vi "PH_USB600x_AnalogReader.ProcCases.vi"(0 "i ref in":refnum<vi>, 1 "selector":string, 2 "Data":T1, 3 "call cluster":T2={"Object"="", "Selector"="", "CallType"=enum."synchronous", "Async Object"="", "Async Selector"="", "Data Descriptor"="", "Data"=[], "Error #"=0, "Expire"=0}, 5 "error in (no error)":errorcluster) -> (14 "i ref out":refnum<vi>, 17 "answer cluster":T2={"Object"="", "Selector"="", "CallType"=enum."synchronous", "Async Object"="", "Async Selector"="", "Data Descriptor"="", "Data"=[], "Error #"=0, "Expire"=0}, 19 "error out":errorcluster)   [LabVIEW 2014, in "PH_USB600x_AnalogReader.lvlib"]
doc: "This method is called by a process from within the default case in the event loop. The methods of a class that are linked to events will be called from THIS method. Add your code here."
uses:
  PH_USB600x_AnalogReader.lvlib
  CS_Core/CSSystem/CoreDefs/CoreDefs.call_type.ctl
  CS_Core/BaseProcess/BaseProcess.descriptor string definition.ctl
  CS_Core/CSSystem/CoreDefs/CoreDefs.rawDataType.ctl
  CS_Core/CSSystem/CoreLib/CoreLib.byte array 2 int.vi
  CS_Core/CSSystem/CoreLib/CoreLib.byte array 2 double.vi
  CS_Core/CSSystem/CoreLib/CoreLib.string 2 byte array.vi
  CS_Core/CSSystem/CoreLib/CoreLib.byte array 2 string.vi
  CS_Core/CSSystem/CoreLib/CoreLib.byte array 2 short.vi
  CS_Core/CSSystem/CoreLib/CoreLib.lvlib
  CS_Core/BaseProcess/BaseProcess.lvlib
  CS_Core/CSApplicationBaseClasses/DeviceBase/DeviceBase.lvlib
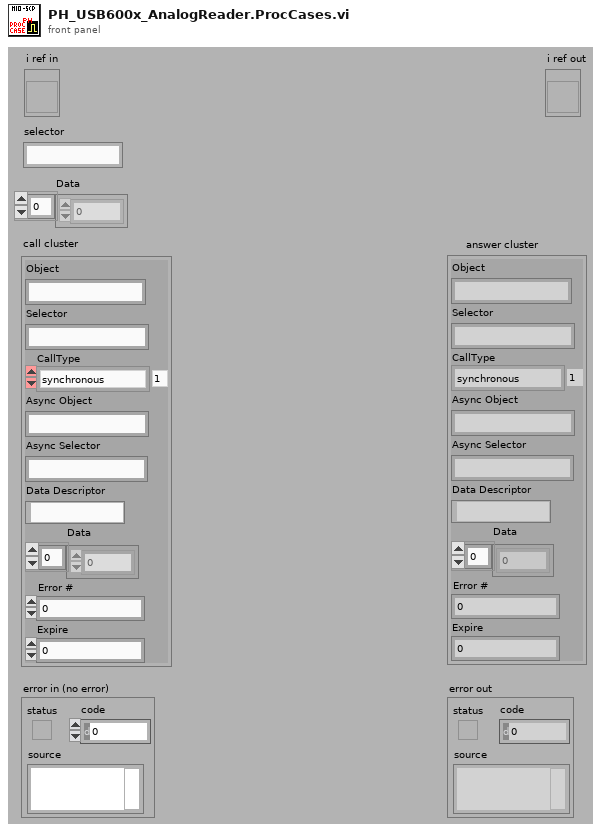
[diagram p1: front panel]
types:
  T1 = typedef "CoreDefs.rawDataType.ctl" = i8[]
  T2 = typedef "CoreDefs.call_type.ctl" = cluster{"Object":string, "Selector":string, "CallType":enum16{"simple", "synchronous", "asynchronous"}, "Async Object":string, "Async Selector":string, "Data Descriptor":T3, "Data":T1, "Error #":i32, "Expire":u32}
  T3 = typedef "BaseProcess.lvlib/BaseProcess.descriptor string definition.ctl" = string
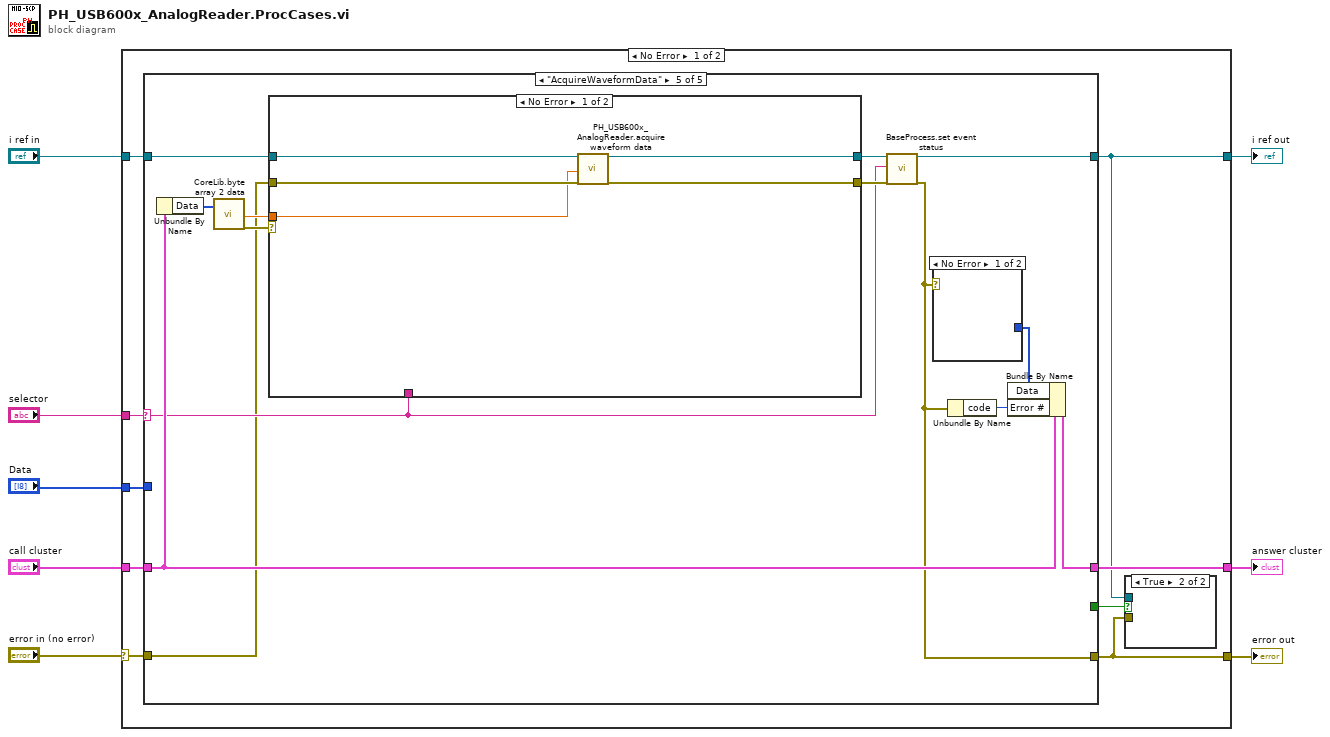
[diagram p0: block diagram]
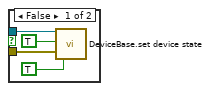
[diagram p2: hidden frame]
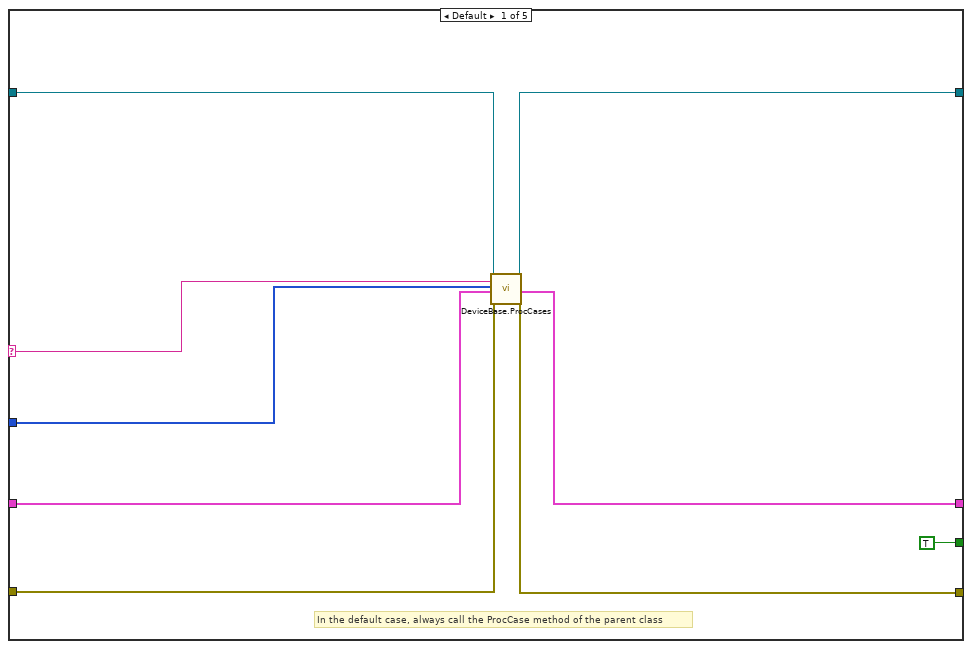
[diagram p3: hidden frame]
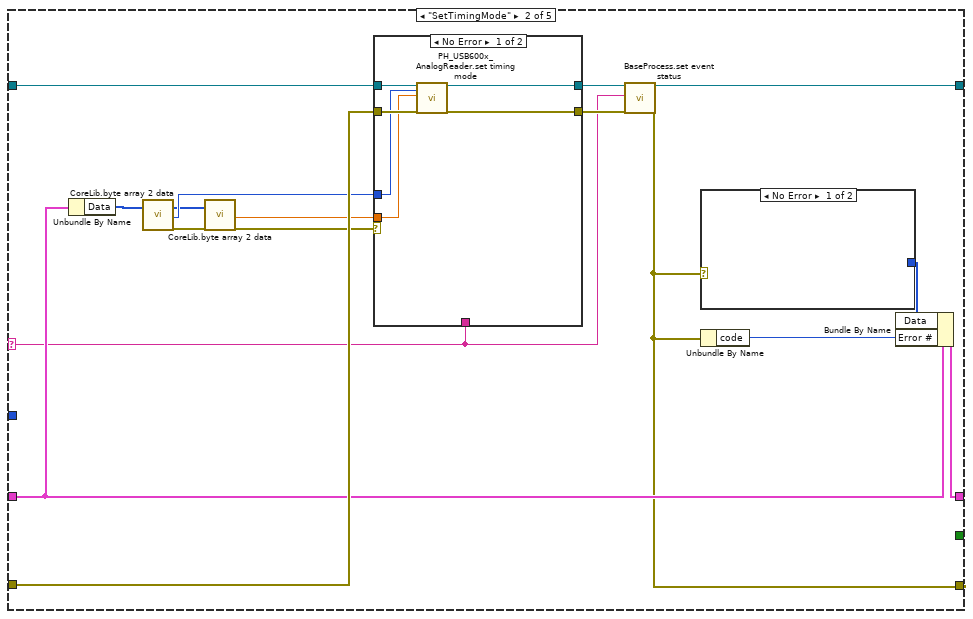
[diagram p4: hidden frame]
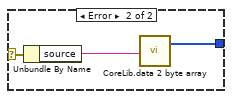
[diagram p5: hidden frame]
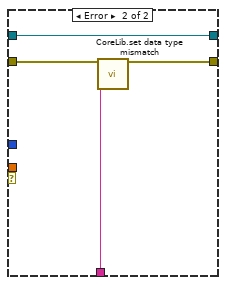
[diagram p6: hidden frame]
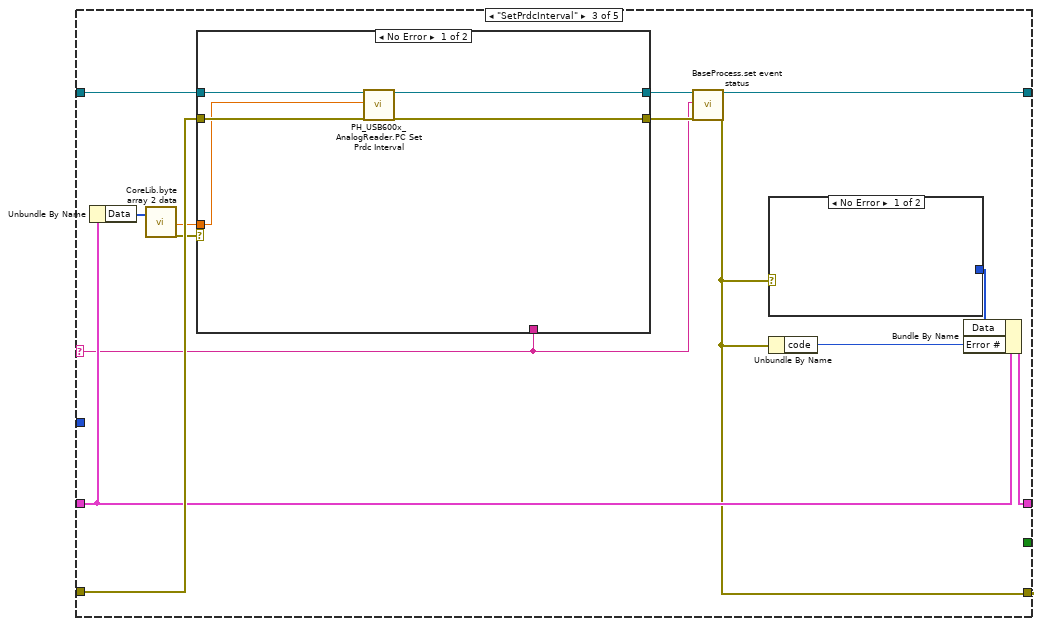
[diagram p7: hidden frame]
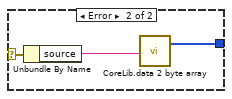
[diagram p8: hidden frame]
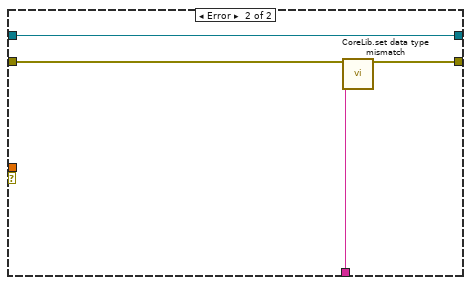
[diagram p9: hidden frame]
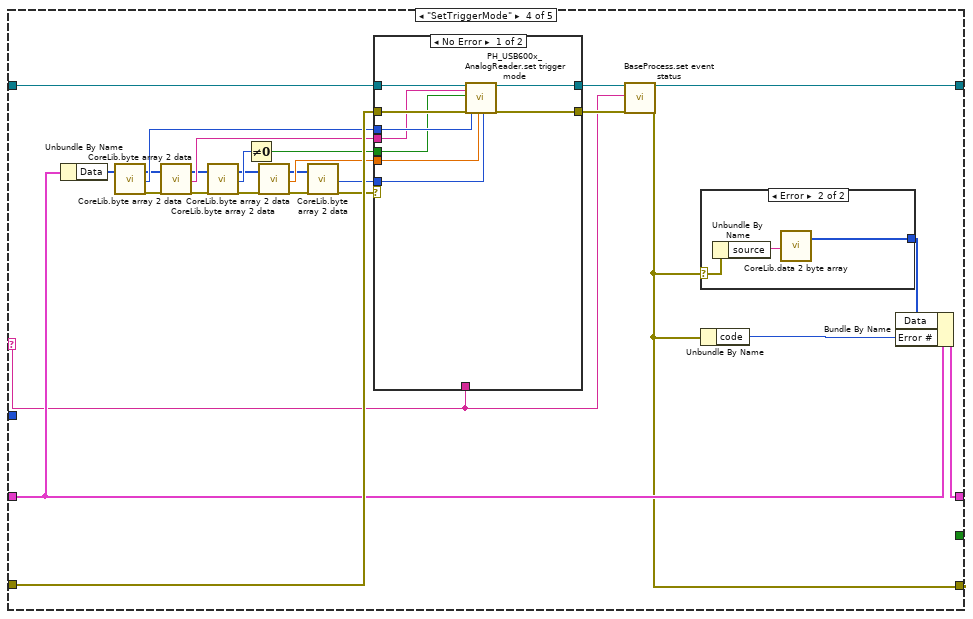
[diagram p10: hidden frame]
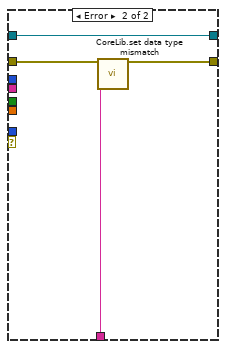
[diagram p12: hidden frame]
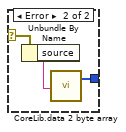
[diagram p13: hidden frame]
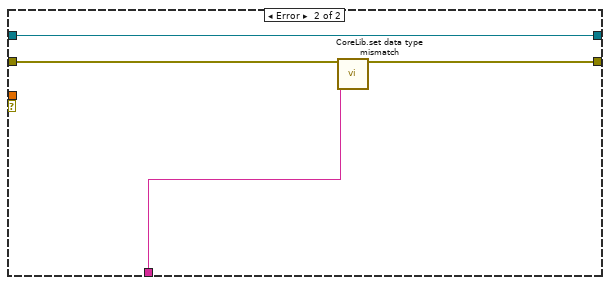
[diagram p14: hidden frame]
diagram:
  n1 = case shown="No Error" "error in (no error)" {
    selector: "error in (no error)" -> [w12 w156]
    tunnel: "selector" -> [w17 _]
    tunnel: [w16 w157] -> w7
    tunnel: "Data" -> [w15 _]
    tunnel: "call cluster" -> [w14 w157]
    tunnel: "i ref in" -> [w13 w158]
    tunnel: [w10 w158] -> w3
    tunnel: [w9 w156] -> w2
    frame No Error {
      n2 = case shown="\"AcquireWaveformData\"" w17 {
        selector: w17 -> [w24 w38 w65 w104 w135]
        tunnel: w15 -> [w25 _ _ _ _]
        tunnel: w13 -> [w23 w47 w74 w113 w143]
        tunnel: [w30 w37 w64 w103 w134] -> w10
        tunnel: w14 -> [w26 w44 w71 w110 w141]
        tunnel: [w27 w43 w70 w109 w140] -> w16
        tunnel: w12 -> [w29 w46 w73 w112 w130]
        tunnel: [w28 w39 w66 w105 w136] -> w9
        tunnel: [TRUE _ _ _ _] -> w11
        frame Default {
          # "In the default case, always call the ProcCase method of the parent class"
          n3 = call "DeviceBase.ProcCases.vi"("i ref in"=w23, "selector"=w24, "Data"=w25, "call cluster"=w26, "error in (no error)"=w29) -> ("i ref out"=w30:refnum<vi>, "answer cluster"=w27:T2, "error out"=w28:errorcluster)  [unwired: 12 in]
        }
        frame "SetTimingMode" {
          n4 = Unbundle By Name(w44) -> ("Data"=w36:T1)
          n5 = call-poly "CoreLib.byte array 2 data.vi"("byteArray"=w36) -> ("byteArray out"=w34:T1, "i32"=w35:i32, "error out"=w32:errorcluster)  [unwired: 16 in]
          n6 = call-poly "CoreLib.byte array 2 data.vi"("byteArray"=w34, "error in (no error)"=w32) -> ("d64"=w33:dbl, "error out"=w31:errorcluster)  [unwired: 15 in, 1 out]
          n7 = case shown="No Error" w31 {
            tunnel: [w51 w60] -> w41
            tunnel: w47 -> [w56 w60]
            tunnel: w46 -> [w55 w59]
            tunnel: [w52 w58] -> w40
            tunnel: w33 -> [w53 _]
            tunnel: w38 -> [_ w57]
            tunnel: w35 -> [w54 _]
            frame No Error {
              n8 = call "PH_USB600x_AnalogReader.set timing mode.vi"("i ref in"=w56, "Samples per Channel"=w54, "Rate"=w53, "error in (no error)"=w55) -> ("i ref out"=w51:refnum<vi>, "error out"=w52:errorcluster)  [unwired: 14 in]
            }
            frame Error {
              n9 = call "CoreLib.set data type mismatch.vi"("error in (no error)"=w59, "error source"=w57) -> ("error out"=w58:errorcluster)  [unwired: 17 in]
            }
          }
          n10 = call "BaseProcess.set event status.vi"("i ref in"=w41, "EventStatus"=w38, "error in (no error)"=w40) -> ("i ref out"=w37:refnum<vi>, "error out"=w39:errorcluster)  [unwired: 14 in, 1 out]
          n11 = case shown="No Error" w39 {
            selector: w39 -> [_ w50]
            tunnel: [_ w48] -> w42
            frame No Error {
            }
            frame Error {
              n12 = Unbundle By Name(w50) -> ("source"=w49:string)
              n13 = call-poly "CoreLib.data 2 byte array.vi"("string"=w49) -> ("byteArray out"=w48:T1)  [unwired: 18 in]
            }
          }
          n14 = Unbundle By Name(w39) -> ("code"=w45:i32)
          n15 = Bundle By Name(cluster=w44, "Data"=w42, "Error #"=w45) -> (w43:T2)
        }
        frame "SetPrdcInterval" {
          n16 = Unbundle By Name(w71) -> ("Data"=w61:T1)
          n17 = call-poly "CoreLib.byte array 2 data.vi"("byteArray"=w61) -> ("d64"=w63:dbl, "error out"=w62:errorcluster)  [unwired: 16 in, 1 out]
          n18 = case shown="No Error" w62 {
            tunnel: [w79 w86] -> w68
            tunnel: w74 -> [w81 w86]
            tunnel: w73 -> [w82 w85]
            tunnel: [w78 w84] -> w67
            tunnel: w63 -> [w80 _]
            tunnel: w65 -> [_ w83]
            frame No Error {
              n19 = call "PH_USB600x_AnalogReader.PC Set Prdc Interval.vi"("i ref in"=w81, "prdc interval [s]"=w80, "error IO"=w82) -> ("i ref out"=w79:refnum<vi>, "error out"=w78:errorcluster)  [unwired: 15 in]
            }
            frame Error {
              n20 = call "CoreLib.set data type mismatch.vi"("error in (no error)"=w85, "error source"=w83) -> ("error out"=w84:errorcluster)  [unwired: 17 in]
            }
          }
          n21 = call "BaseProcess.set event status.vi"("i ref in"=w68, "EventStatus"=w65, "error in (no error)"=w67) -> ("i ref out"=w64:refnum<vi>, "error out"=w66:errorcluster)  [unwired: 14 in, 1 out]
          n22 = case shown="No Error" w66 {
            selector: w66 -> [_ w77]
            tunnel: [_ w75] -> w69
            frame No Error {
            }
            frame Error {
              n23 = Unbundle By Name(w77) -> ("source"=w76:string)
              n24 = call-poly "CoreLib.data 2 byte array.vi"("string"=w76) -> ("byteArray out"=w75:T1)  [unwired: 18 in]
            }
          }
          n25 = Unbundle By Name(w66) -> ("code"=w72:i32)
          n26 = Bundle By Name(cluster=w71, "Data"=w69, "Error #"=w72) -> (w70:T2)
        }
        frame "SetTriggerMode" {
          n27 = Unbundle By Name(w110) -> ("Data"=w102:T1)
          n28 = call-poly "CoreLib.byte array 2 data.vi"("byteArray"=w102) -> ("byteArray out"=w100:T1, "i32"=w101:i32, "error out"=w99:errorcluster)  [unwired: 16 in]
          n29 = call-poly "CoreLib.byte array 2 data.vi"("byteArray"=w100, "error in (no error)"=w99) -> ("byteArray out"=w97:T1, "string"=w98:string, "error out"=w96:errorcluster)  [unwired: 15 in]
          n30 = call-poly "CoreLib.byte array 2 data.vi"("byteArray"=w97, "error in (no error)"=w96) -> ("byteArray out"=w93:T1, "i16"=w95:i16, "error out"=w92:errorcluster)  [unwired: 15 in]
          n31 = Not Equal To 0?(x=w95) -> (x != 0?=w94:bool)
          n32 = call-poly "CoreLib.byte array 2 data.vi"("byteArray"=w93, "error in (no error)"=w92) -> ("byteArray out"=w90:T1, "d64"=w91:dbl, "error out"=w89:errorcluster)  [unwired: 15 in]
          n33 = call-poly "CoreLib.byte array 2 data.vi"("byteArray"=w90, "error in (no error)"=w89) -> ("i32"=w88:i32, "error out"=w87:errorcluster)  [unwired: 15 in, 1 out]
          n34 = case shown="No Error" w87 {
            tunnel: [w124 w129] -> w107
            tunnel: w113 -> [w125 w129]
            tunnel: w112 -> [w123 w128]
            tunnel: [w122 w127] -> w106
            tunnel: w98 -> [w120 _]
            tunnel: w104 -> [_ w126]
            tunnel: w101 -> [w121 _]
            tunnel: w94 -> [w119 _]
            tunnel: w91 -> [w118 _]
            tunnel: w88 -> [w117 _]
            frame No Error {
              n35 = call "PH_USB600x_AnalogReader.set trigger mode.vi"("i ref in"=w125, "triggerSource (\"PFI0\")"=w120, "edgeRising"=w119, "error in (no error)"=w123, "triggerType"=w121, "level"=w118, "pretriggerSamples"=w117) -> ("i ref out"=w124:refnum<vi>, "error out"=w122:errorcluster)  [unwired: 11 in]
            }
            frame Error {
              n36 = call "CoreLib.set data type mismatch.vi"("error in (no error)"=w128, "error source"=w126) -> ("error out"=w127:errorcluster)  [unwired: 17 in]
            }
          }
          n37 = call "BaseProcess.set event status.vi"("i ref in"=w107, "EventStatus"=w104, "error in (no error)"=w106) -> ("i ref out"=w103:refnum<vi>, "error out"=w105:errorcluster)  [unwired: 14 in, 1 out]
          n38 = case shown="Error" w105 {
            selector: w105 -> [_ w116]
            tunnel: [_ w114] -> w108
            frame No Error {
            }
            frame Error {
              n39 = Unbundle By Name(w116) -> ("source"=w115:string)
              n40 = call-poly "CoreLib.data 2 byte array.vi"("string"=w115) -> ("byteArray out"=w114:T1)  [unwired: 18 in]
            }
          }
          n41 = Unbundle By Name(w105) -> ("code"=w111:i32)
          n42 = Bundle By Name(cluster=w110, "Data"=w108, "Error #"=w111) -> (w109:T2)
        }
        frame "AcquireWaveformData" {
          n43 = Unbundle By Name(w141) -> ("Data"=w133:T1)
          n44 = call-poly "CoreLib.byte array 2 data.vi"("byteArray"=w133) -> ("d64"=w132:dbl, "error out"=w131:errorcluster)  [unwired: 16 in, 1 out]
          n45 = case shown="No Error" w131 {
            tunnel: [w151 w155] -> w138
            tunnel: w143 -> [w148 w155]
            tunnel: w130 -> [w149 w154]
            tunnel: [w150 w153] -> w137
            tunnel: w135 -> [_ w152]
            tunnel: w132 -> [w147 _]
            frame No Error {
              n46 = call "PH_USB600x_AnalogReader.acquire waveform data.vi"("i ref in"=w148, "Device Timeout [sec] (1)"=w147, "error in (no error)"=w149) -> ("i ref out"=w151:refnum<vi>, "error out"=w150:errorcluster)  [unwired: 15 in]
            }
            frame Error {
              n47 = call "CoreLib.set data type mismatch.vi"("error in (no error)"=w154, "error source"=w152) -> ("error out"=w153:errorcluster)  [unwired: 17 in]
            }
          }
          n48 = call "BaseProcess.set event status.vi"("i ref in"=w138, "EventStatus"=w135, "error in (no error)"=w137) -> ("i ref out"=w134:refnum<vi>, "error out"=w136:errorcluster)  [unwired: 14 in, 1 out]
          n49 = case shown="No Error" w136 {
            selector: w136 -> [_ w146]
            tunnel: [_ w144] -> w139
            frame No Error {
            }
            frame Error {
              n50 = Unbundle By Name(w146) -> ("source"=w145:string)
              n51 = call-poly "CoreLib.data 2 byte array.vi"("string"=w145) -> ("byteArray out"=w144:T1)  [unwired: 18 in]
            }
          }
          n52 = Unbundle By Name(w136) -> ("code"=w142:i32)
          n53 = Bundle By Name(cluster=w141, "Data"=w139, "Error #"=w142) -> (w140:T2)
        }
      }
      n54 = case shown="True" w11 {
        tunnel: w10 -> [w21 _]
        tunnel: w9 -> [w20 _]
        frame False {
          n55 = call "DeviceBase.set device state.vi"("i ref in"=w21, "implicit"=TRUE, "device error"=w20, "mayResetError (FALSE)"=TRUE) -> ()  [unwired: 13 in, 3 out]
        }
        frame True {
        }
      }
    }
    frame Error {
    }
  }
  "answer cluster" <- w7
  "i ref out" <- w3
  "error out" <- w2
